vi "Sample Out.vi"(8 "error in (no error)":errorcluster, 11 "CO2 Actor in":refnum<class "CO2 Actor.lvclass">) -> (0 "error out":errorcluster, 3 "CO2 Actor out":refnum<class "CO2 Actor.lvclass">)   [LabVIEW 2015, in "cRIO-Carbondioxide.lvlib" / "CO2-Actor.lvlib" / "CO2 Actor.lvclass"]
uses:
  CO2 Actor.lvclass
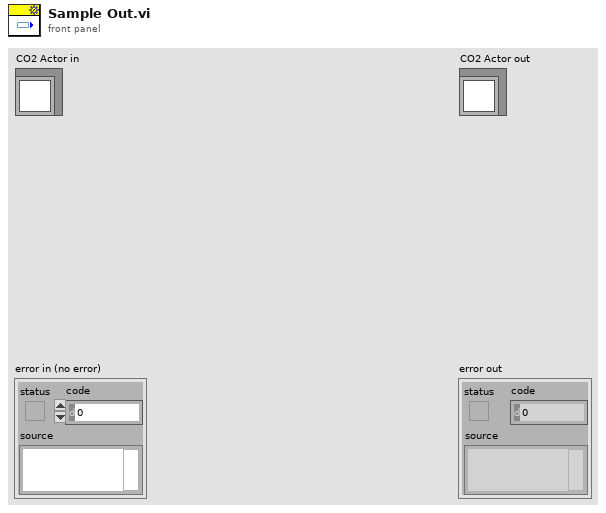
[diagram p1: front panel]
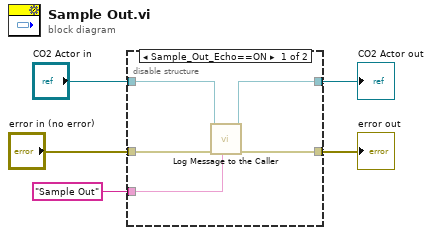
[diagram p0: block diagram]
diagram:
  n1 = disable-structure shown="Sample_Out_Echo==ON" {
    disable-tunnel: "error in (no error)" -> [w10 w11]
    disable-tunnel: [w9 w11] -> w4
    disable-tunnel: "Sample Out" ("String (\"OK\")") -> [w8 _]
    disable-tunnel: "CO2 Actor in" -> [w7 w12]
    disable-tunnel: [w6 w12] -> w1
    frame condition #0 {
      n2 = call-dynamic "Log Message to the Caller.vi"("String (\"\" = no message to send)"=w8, "error in (no error)"=w10, "CO2 Actor in"=w7) -> ("error out"=w9:errorcluster, "CO2 Actor out"=w6:refnum<class "CO2 Actor.lvclass">)  [unwired: 7 in]
    }
    frame condition #1 (active) {
    }
  }
  "error out" <- w4
  "CO2 Actor out" <- w1
